vi "ManualTresholdControlNOGENASICTESt.vi"() -> ()   [LabVIEW 2012]
uses:
  <vilib>/Utility/NIReport.llb/NI_report.lvclass
  <vilib>/Utility/NIReport.llb/HTML/NI_HTML.lvclass
panel:
  in  "Att gain":u32=15
  in  "IPR?":bool
  out "Data":string="empty_read_buffer0_2-65@1\r\n0_2-75@0\r\n"
  out "IPR_count":u32
  in  "Channel":i8
  in  "Instrument VISA in":T1={"AWG VISA"="AgilentGenerator1", "Oscilloscope  VISA "="AgilentOsciloscope", "Integration Board IP"="172.16.17.47", "connection ID"=refnum, "report out"=refnum, "report file path"=path "C:/Documents and Settings/CTA_LAB01/Desktop/L0_Asic/L0 Asic Test Data"}
  in  "Treshold":i16=542 min=0 max=1000
  in  "stop":bool
  out "error out":errorcluster
  in  "error in":errorcluster
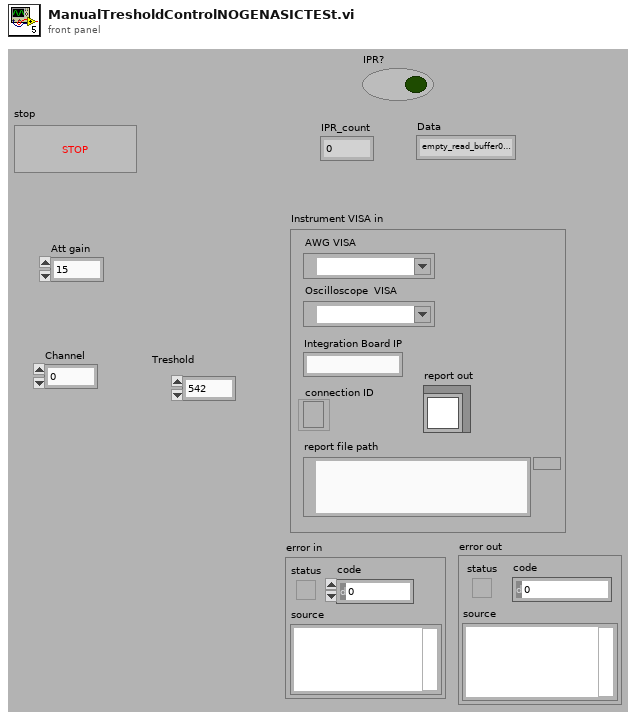
[diagram p1: front panel]
types:
  T1 = cluster{"AWG VISA":refnum<visa-resource-name>, "Oscilloscope  VISA ":refnum<visa-resource-name>, "Integration Board IP":string, "connection ID":refnum<k5>, "report out":refnum<class "NI_report.lvclass">, "report file path":path}
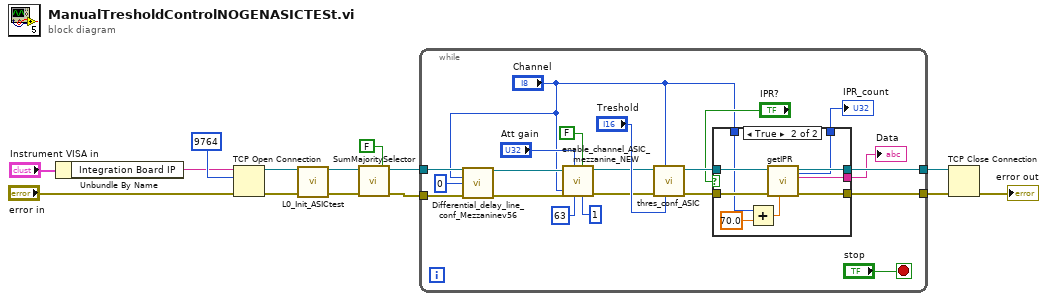
[diagram p0: block diagram]
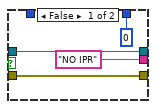
[diagram p2: hidden frame]
diagram:
  n1 = Unbundle By Name("Instrument VISA in") -> ("Integration Board IP"=w9:string)
  n2 = TCP Open Connection(address=w9, remote port or service name=u16 9764, error in (no error)="error in") -> (connection ID=w2:refnum<k5>, error out=w3:errorcluster)  [unwired: 2 in]
  n3 = call "L0_Init_ASICtest.vi"("error in"=w3, "connection ID in"=w2) -> ("error out"=w4:errorcluster, "connection ID out"=w1:refnum<k5>)  [unwired: 8 in]
  n4 = call "SumMajoritySelector.vi"("On Sum\nOff Majority"=FALSE ("On Sum\nOff Majority"), "error in (no error)"=w4, "connection ID"=w1) -> ("error out"=w7:errorcluster, "connection ID out"=w8:refnum<k5>)  [unwired: 5 in]
  n5 = while {
    tunnel: [w27] -> w12
    tunnel: [w25] -> w11
    tunnel: w7 -> [w20]
    tunnel: w8 -> [w18]
    stop <- "stop" stop-if-true
    n6 = call "Differential_delay_line_conf_Mezzaninev56.vi"("connection ID"=w18, "channel"="Channel", "Delay value"=u16 0, "error in (no error)"=w20) -> ("connection ID out"=w17:refnum<k5>, "error out 2"=w19:errorcluster)  [unwired: 4 in, 6 out]
    n7 = call "enable_channel_ASIC_mezzanine_NEW.vi"("Clip_sel_b"=u32 1, "maj/sum"=FALSE, "Ib_clipVb"=u32 63, "Att gain"="Att gain", "error in"=w19, "Channel"="Channel", "connection ID"=w17) -> ("error out"=w33:errorcluster, "connection ID out"=w32:refnum<k5>)  [unwired: 2 in, 1 out]
    n8 = call "thres_conf_ASIC.vi"("threshold"="Treshold", "Ring"="Channel", "error out 3"=w33, "connection ID"=w32) -> ("error out 2"=w28:errorcluster, "connection ID out"=w26:refnum<k5>)  [unwired: 4 in, 2 out]
    n9 = case shown="True" "IPR?" {
      tunnel: w28 -> [w39 w48]
      tunnel: [w39 w47] -> w27
      tunnel: w26 -> [w38 w46]
      tunnel: [w38 w45] -> w25
      tunnel: "Channel" -> [_ w42]
      tunnel: [u32 0 ("IPR_count") w41] -> w24
      tunnel: ["NO IPR" ("Data") w40] -> w23
      frame False {
      }
      frame True {
        n10 = Add(x=w42, y=70.0) -> (x+y=w44:dbl)
        n11 = call "getIPR.vi"("Address"=w44, "error in"=w48, "connection ID"=w46) -> ("error out"=w47:errorcluster, "Data"=w40:string, "connection ID out"=w45:refnum<k5>, "IPR_count"=w41:u32)  [unwired: 5 in]
      }
    }
    "IPR_count" <- w24
    "Data" <- w23
  }
  n12 = TCP Close Connection(connection ID=w11, error in (no error)=w12) -> (error out=→"error out":errorcluster)  [unwired: 1 in, 1 out]
